vi "CheckSRsStatus(SubVI).vi"(8 "Error In":errorcluster, 9 "Statuses":string[](array[string]), 10 "Period":T1={"Start Date"=timestamp(-113047311.23669147 s since 1904-01-01), "End Date"=timestamp(9354056288.76331 s since 1904-01-01)}, 11 "Report Data In":T2[](array[typedef])) -> (0 "Error Out":errorcluster, 3 "SR Data Out":T3[](array[typedef]))   [LabVIEW 2017, in "DS_Lib.lvlib" / "SRReportParser.lvlib"]
uses:
  SRReportParser.lvlib
  TypeDefs/InWorkSR_Data.ctl
  Modules/Private Controls/Data Raw.ctl
  Modules/Data Operations.lvlib
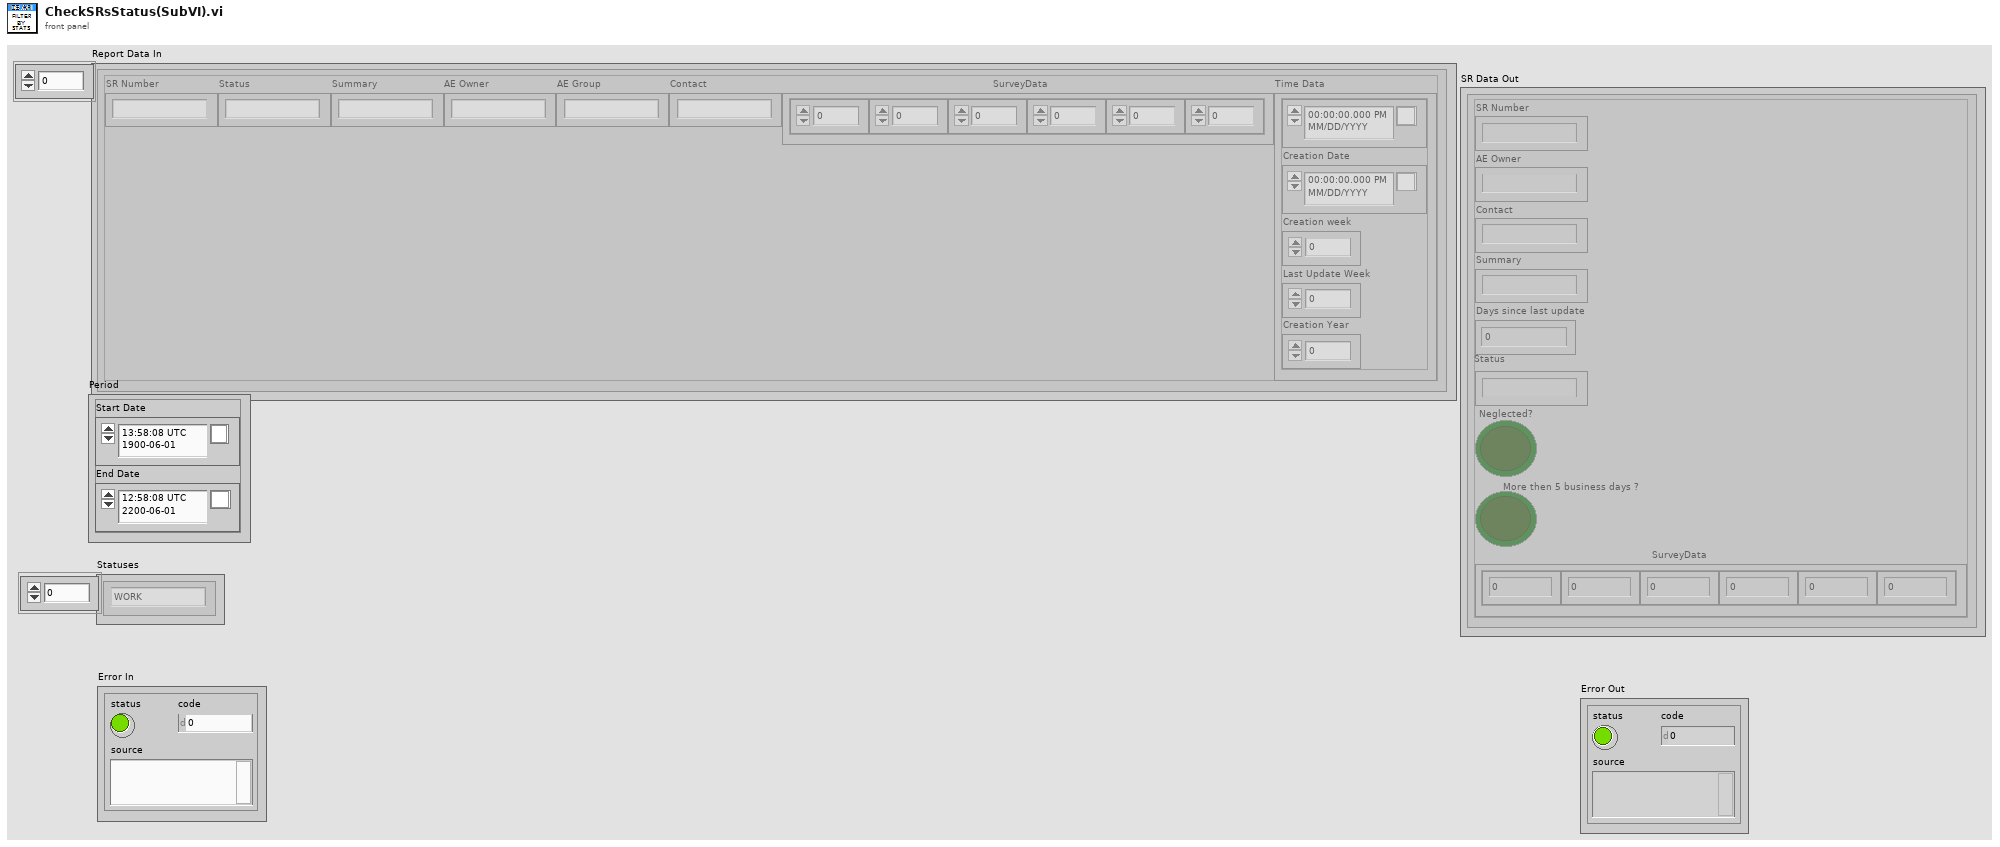
[diagram p1: front panel]
types:
  T1 = cluster{"Start Date":timestamp, "End Date":timestamp}
  T2 = typedef "Data Operations.lvlib/Data Raw.ctl" = cluster{"SR Number":string, "Status":string, "Summary":string, "AE Owner":string, "AE Group":string, "Contact":string, "SurveyData":cluster{"Resolution Time":dbl, "Total Satisfaction":dbl, "Response Time":dbl, "Courtesy":dbl, "Problem Solved":dbl, "Level of effort":dbl}, "Time Data":cluster{"Last Update Date":timestamp, "Creation Date":timestamp, "Creation week":i16, "Last Update Week":i16, "Creation Year":i16}}
  T3 = typedef "DS_Lib.lvlib/SRReportParser.lvlib/InWorkSR_Data.ctl" = cluster{"SR Number":string, "AE Owner":string, "Contact":string, "Summary":string, "Days since last update":dbl, "Status":string, "Neglected?":bool, "More then 5 business days ?":bool, "SurveyData":cluster{"Resolution Time":dbl, "Total Satisfaction":dbl, "Response Time":dbl, "Courtesy":dbl, "Problem Solved":dbl, "Level of effort":dbl}}
  T4 = cluster{"Resolution Time":dbl, "Total Satisfaction":dbl, "Response Time":dbl, "Courtesy":dbl, "Problem Solved":dbl, "Level of effort":dbl}
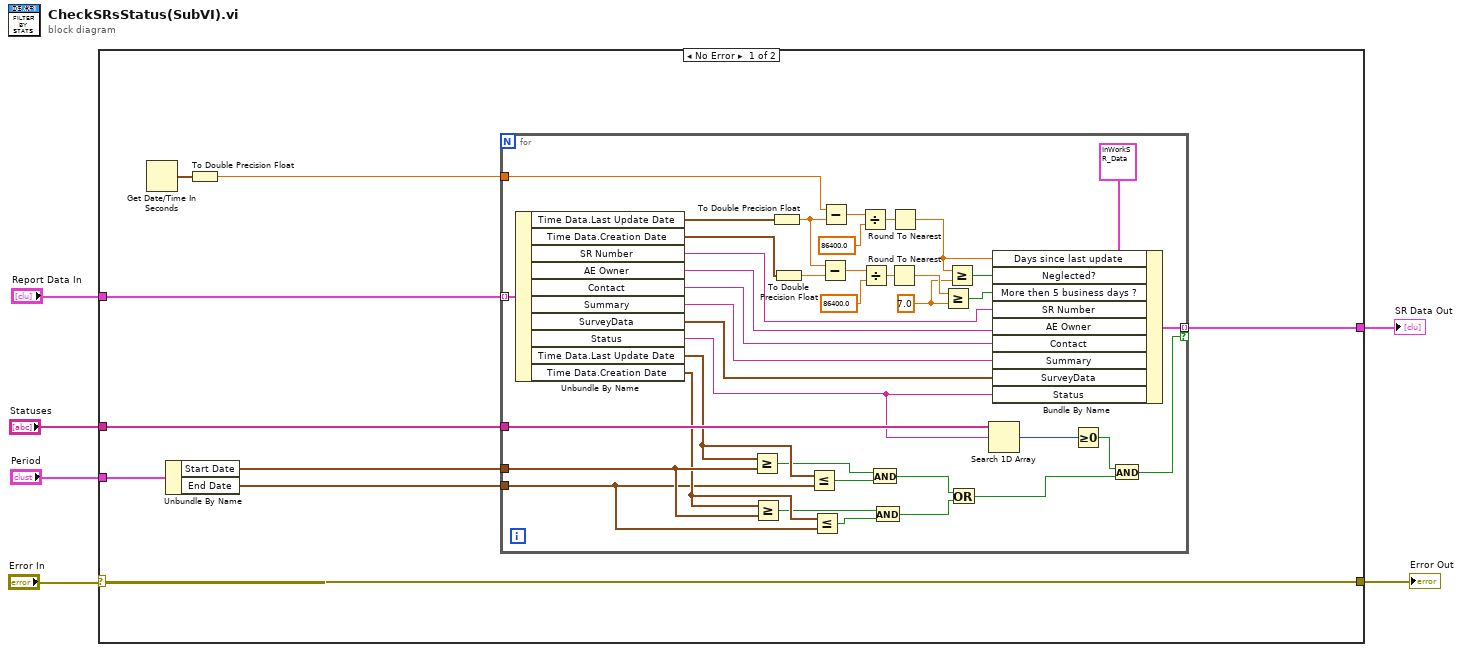
[diagram p0: block diagram]
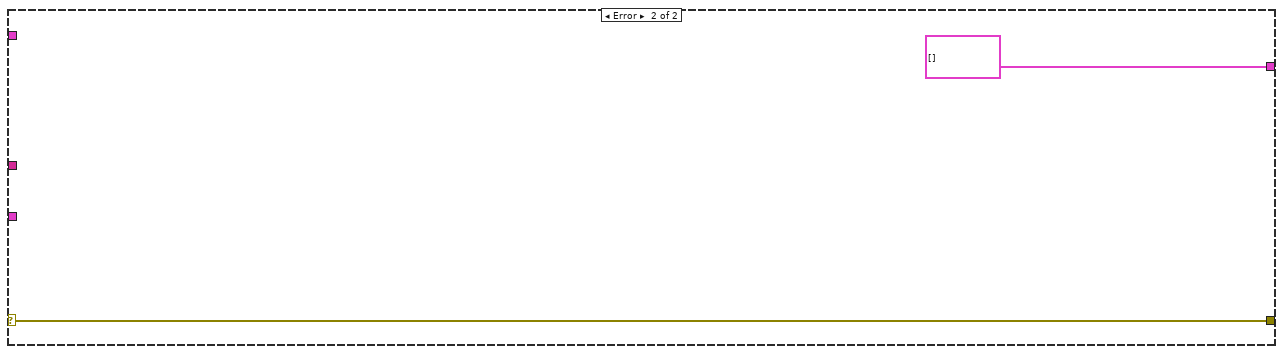
[diagram p2: hidden frame]
diagram:
  n1 = case shown="No Error" "Error In" {
    selector: "Error In" -> [w14 w57]
    tunnel: [w7 T3[] []] -> w6
    tunnel: "Report Data In" -> [w15 _]
    tunnel: [w14 w57] -> w3
    tunnel: "Statuses" -> [w13 _]
    tunnel: "Period" -> [w12 _]
    frame No Error {
      n2 = Get Date/Time In Seconds() -> (seconds since 1Jan1904=w9:timestamp)
      n3 = Unbundle By Name(w12) -> ("Start Date"=w11:timestamp, "End Date"=w10:timestamp)
      n4 = To Double Precision Float(number=w9) -> (double precision float=w8:dbl)
      n5 = for {
        tunnel: w15 -> [w55] mode=indexing
        tunnel: [w42] -> w7 mode=indexing if=w40
        tunnel: w13 -> [w30]
        tunnel: w11 -> [w23]
        tunnel: w10 -> [w21]
        tunnel: w8 -> [w38]
        w32 = 7.0 ("y")
        n6 = Unbundle By Name(w55) -> ("Time Data.Last Update Date"=w39:timestamp, "Time Data.Creation Date"=w53:timestamp, "SR Number"=w46:string, "AE Owner"=w45:string, "Contact"=w44:string, "Summary"=w43:string, "SurveyData"=w41:T4, "Status"=w29:string, "Time Data.Last Update Date"=w26:timestamp, "Time Data.Creation Date"=w22:timestamp)
        n7 = Greater Or Equal?(x=w26, y=w23) -> (x >= y?=w25:bool)
        n8 = Greater Or Equal?(x=w22, y=w23) -> (x >= y?=w20:bool)
        n9 = To Double Precision Float(number=w39) -> (double precision float=w37:dbl)
        n10 = To Double Precision Float(number=w53) -> (double precision float=w54:dbl)
        n11 = Less Or Equal?(x=w26, y=w21) -> (x <= y?=w24:bool)
        n12 = Less Or Equal?(x=w22, y=w21) -> (x <= y?=w19:bool)
        n13 = Subtract(x=w37, y=w54) -> (x-y=w52:dbl)
        n14 = Subtract(x=w38, y=w37) -> (x-y=w35:dbl)
        n15 = Divide(x=w35, y=86400.0) -> (x/y=w34:dbl)
        n16 = Divide(x=w52, y=86400.0) -> (x/y=w49:dbl)
        n17 = And(x=w25, y=w24) -> (x .and. y?=w18:bool)
        n18 = And(x=w20, y=w19) -> (x .and. y?=w17:bool)
        n19 = Round To Nearest(number=w49) -> (nearest integer value=w48:dbl)
        n20 = Round To Nearest(number=w34) -> (nearest integer value=w31:dbl)
        n21 = Greater Or Equal?(x=w48, y=w32) -> (x >= y?=w47:bool)
        n22 = Greater Or Equal?(x=w31, y=w32) -> (x >= y?=w33:bool)
        n23 = Or(x=w18, y=w17) -> (x .or. y?=w16:bool)
        n24 = Search 1D Array(1D array=w30, element=w29) -> (index of element=w27:i32)  [unwired: 1 in]
        n25 = Bundle By Name(cluster=T3 {"SR Number"="", "AE Owner"="", "Contact"="", "Summary"="", "Days since last update"=0.0, "Status"="", "Neglected?"=FALSE, "More then 5 business days ?"=FALSE, "SurveyData"={"Resolution Time"=0.0, "Total Satisfaction"=0.0, "Response Time"=0.0, "Courtesy"=0.0, "Problem Solved"=0.0, "Level of effort"=0.0}}, "Days since last update"=w31, "Neglected?"=w33, "More then 5 business days ?"=w47, "SR Number"=w46, "AE Owner"=w45, "Contact"=w44, "Summary"=w43, "SurveyData"=w41, "Status"=w29) -> (w42:T3)
        n26 = Greater Or Equal To 0?(x=w27) -> (x >= 0?=w28:bool)
        n27 = And(x=w28, y=w16) -> (x .and. y?=w40:bool)
      }
    }
    frame Error {
    }
  }
  "SR Data Out" <- w6
  "Error Out" <- w3
